vi "p2.vi"() -> ()   [LabVIEW 2021, in "d9.lvlib"]
uses:
  d9.lvlib
  939e70a1-15eb-480c-88e0-20e72bed207b.vi
  AOC/AOC.lvlib
panel:
  in  "Defer Panel Updates":bool=TRUE
  in  "Move Delay":u32
  out "Moves Remaining":i32
  out "Rope":cluster{"x":i64, "y":i64}[](graph)
  in  "Example":string="R 5\nU 8\nL 8\nD 3\nR 17\nD 10\nL 25\nU 20"
  in  "Example":bool=TRUE
  out "Answer":i32=36
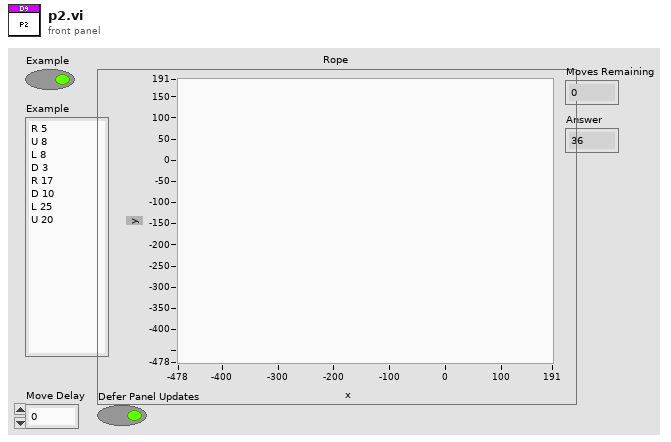
[diagram p1: front panel]
diagram:
  w3 = -10.0 ("X Scale.Range:Minimum")
  w4 = 10.0 ("X Scale.Range:Maximum")
  w8 = 10 ("dimension size")
  n1 = control-ref of="Rope"() -> (w6:refnum<vi>)
  n2 = property on="Property Node" class="XYGraph (strict)"(reference=w6, "XScale.Maximum"=w4, "YScale.Maximum"=w4, "XScale.Minimum"=w3, "YScale.Minimum"=w3) -> (reference out=w5:refnum<vi>)  [unwired: 1 in, 1 out]
  n3 = call "Get Input.vi"() -> ()  [unwired: 11 in, 1 out]
  n4 = Select(t="Example", s="Example", f="R 1\nU 2\nR 1\nL 2\nD 2\nU 1\nR 2\nU 1\nL 2\nU 1\nD 2\nR 1\nD 1\nL 1\nU 2\nD 2\nL 2\nD 1\nU 2\nD 2\nL 1\nU 1\nL 2\nD 2\nU 2\nL 1\nU 2\nL 1\nR 2\nU 1\nL 1\nR 2\nD 1\nU 2\nR 1\nU 1\nR 2\nU 1\nR 2\nU 1\nD 1\nU 1\nD 1\nL 2\nD 2\nR 1\nU 1\nR 1\nU 1\nL 1\nU 1\nD 2\nR 2\nD 2\nL 2\nU 2\nR 1\nD 1\nU 1\nD 2\nR 1\nD 2\nL 2\nR 2\nL 1\nU 1\nL 2\nD 2\nL 2\nD 1\nR 1\nL 2\nD 2\nR 1\nL 1\nR 1\nD 1\nR 1\nD 2\nL 2\nU 1\nD 2\nR 2\nD 1\nU 1\nL 1\nD 1\nU 2\nR 1\nU 1\nL 2\nU 1\nL 1\nU 2\nL 2\nD 2\nU 1\nL 1\nU 2\nD 2\nL 2\nD 2\nR 2\nU 2\nL 2\nD 1\nU 1\nR 2\nD 2\nL 2\nR 2\nD 2\nL 1\nD 1\nU 2\nR 2\nD 3\nR 1\nU 3\nL 3\nD 2\nR 1\nD 1\nL 2\nD 1\nR 2\nU 3\nL 2\nU 2\nR 3\nU 3\nL 1\nD 3\nR 3\nU 2\nR 3\nU 3\nL 1\nD 3\nR 3\nL 2\nR 2\nL 3\nD 3\nR 2\nD 2\nR 2\nD 1\nR 1\nL 1\nD 2\nR 1\nD 2\nU 1\nR 2\nL 2\nR 2\nU 2\nR 2\nD 1\nU 1\nD 1\nL 3\nU 3\nD 3\nL 1\nU 2\nR 2\nU 2\nR 1\nU 1\nL 2\nU 2\nR 3\nU 1\nD 3\nR 3\nU 2\nR 1\nU 1\nD 3\nL 2\nU 3\nL 1\nR 2\nD 3\nR 2\nU 1\nR 2\nD 1\nU 3\nL 2\nD 1\nR 1\nL 3\nR 3\nD 2\nR 1\nU 2\nR 3\nD 2\nU 2\nL 2\nU 1\nR 2\nU 2\nL 2\nD 3\nL 2\nD 1\nL 1\nU 2\nL 1\nD 2\nR 1\nD 2\nR 1\nL 2\nU 1\nL 1\nU 1\nD 2\nR 4\nD 4\nL 2\nR 4\nD 1\nL 2\nD 2\nL 4\nU 4\nD 4\nL 3\nR 3\nD 1\nL 1\nD 1\nU 4\nR 4\nU 4\nD 2\nR 1\nU 3\nR 2\nU 3\nR 4\nD 3\nU 3\nL 4\nD 1\nR 2\nU 3\nD 4\nU 3\nR 2\nL 1\nD 2\nU 2\nR 3\nU 2\nR 2\nD 2\nL 2\nU 4\nR 1\nL 3\nR 1\nL 1\nD 3\nR 4\nD 2\nR 4\nU 3\nL 1\nD 1\nR 4\nU 3\nD 1\nL 3\nR 1\nL 3\nD 2\nL 2\nR 3\nL 4\nD 4\nU 1\nL 1\nR 1\nD 3\nL 2\nR 1\nD 3\nR 2\nD 4\nU 4\nR 3\nU 1\nD 3\nL 3\nD 3\nU 1\nD 2\nU 4\nR 4\nU 2\nD 1\nR 1\nD 4\nL 2\nR 3\nU 4\nL 1\nD 1\nU 4\nL 3\nD 4\nU 2\nR 4\nU 2\nR 4\nU 2\nL 1\nR 1\nL 3\nD 4\nL 2\nR 2\nL 3\nU 3\nR 4\nL 2\nR 1\nD 5\nU 1\nR 1\nU 2\nR 1\nU 4\nL 3\nU 4\nR 2\nD 3\nL 4\nR 3\nL 2\nU 2\nR 1\nL 3\nD 5\nR 3\nL 2\nU 5\nR 2\nU 5\nL 5\nU 4\nR 4\nD 2\nR 4\nD 3\nR 2\nD 3\nU 2\nL 3\nD 3\nL 1\nU 4\nD 3\nL 1\nD 1\nR 2\nL 4\nR 3\nU 1\nR 3\nL 2\nR 3\nD 4\nR 2\nU 3\nL 4\nR 5\nL 1\nU 1\nD 5\nU 2\nR 5\nL 4\nD 3\nL 1\nD 3\nU 1\nR 2\nD 1\nL 5\nD 2\nR 4\nL 1\nD 2\nR 4\nL 3\nR 3\nL 3\nR 4\nL 3\nU 3\nD 4\nU 2\nR 1\nD 1\nU 1\nR 5\nD 5\nL 5\nR 3\nU 2\nD 4\nL 5\nD 1\nL 4\nR 4\nU 2\nL 2\nR 2\nU 3\nL 1\nU 3\nL 1\nD 4\nU 5\nD 5\nR 4\nL 4\nR 5\nD 4\nU 5\nL 4\nU 1\nD 4\nR 5\nD 2\nU 4\nR 2\nU 3\nD 2\nU 6\nD 4\nR 1\nD 4\nR 3\nL 1\nR 5\nU 6\nD 5\nL 4\nR 3\nL 4\nR 5\nD 1\nR 3\nD 2\nL 6\nU 5\nR 6\nL 2\nD 6\nU 1\nL 3\nD 4\nR 6\nD 3\nL 3\nR 5\nU 6\nD 5\nU 1\nR 4\nL 4\nU 4\nR 5\nD 1\nL 4\nU 6\nL 2\nR 3\nL 2\nR 3\nL 3\nR 4\nU 3\nD 1\nR 6\nD 5\nL 2\nR 4\nU 4\nD 2\nL 1\nR 2\nD 3\nL 4\nD 4\nR 4\nD 6\nR 1\nL 2\nR 5\nD 3\nU 5\nR 4\nL 6\nD 6\nU 4\nR 4\nL 4\nU 4\nR 5\nD 1\nU 1\nR 4\nL 2\nU 6\nD 3\nL 3\nU 6\nD 1\nU 4\nD 6\nR 6\nU 1\nR 2\nU 5\nD 4\nL 2\nU 5\nD 1\nL 5\nU 1\nR 3\nD 2\nR 1\nL 3\nD 1\nR 1\nL 2\nR 6\nD 6\nR 4\nU 4\nL 5\nR 6\nL 5\nR 4\nD 3\nL 2\nR 4\nL 2\nU 6\nD 5\nR 1\nL 3\nR 1\nU 2\nR 6\nL 2\nD 7\nL 2\nD 4\nR 2\nU 6\nD 4\nR 5\nU 6\nR 3\nL 3\nU 2\nR 3\nU 1\nR 7\nU 2\nR 2\nD 7\nR 1\nU 5\nD 1\nL 5\nU 5\nR 2\nD 5\nR 4\nU 5\nL 3\nD 4\nL 6\nR 7\nL 2\nD 3\nL 2\nD 6\nU 6\nL 1\nD 7\nU 6\nL 7\nR 5\nL 1\nU 7\nR 1\nL 4\nR 4\nL 5\nU 7\nD 4\nR 7\nL 5\nU 7\nL 6\nU 3\nD 5\nR 5\nU 7\nR 5\nL 3\nU 6\nR 2\nU 3\nR 3\nU 6\nL 5\nD 6\nL 4\nD 5\nR 1\nL 3\nU 6\nR 6\nU 6\nL 1\nD 2\nL 5\nD 1\nL 6\nU 5\nD 5\nR 5\nD 6\nL 4\nU 5\nR 2\nU 4\nD 7\nL 1\nU 1\nD 1\nL 1\nD 4\nU 1\nL 6\nU 1\nR 5\nD 1\nU 1\nR 1\nU 5\nR 4\nU 5\nL 2\nU 6\nL 7\nR 2\nU 4\nR 5\nL 1\nR 8\nL 2\nD 7\nR 7\nD 2\nL 2\nR 2\nD 2\nU 7\nD 7\nR 4\nU 1\nR 2\nL 6\nU 1\nL 3\nU 2\nD 7\nR 6\nL 5\nD 1\nL 3\nU 6\nD 2\nU 2\nR 4\nD 1\nL 7\nU 3\nD 8\nU 4\nD 8\nL 8\nU 6\nL 3\nU 4\nR 4\nU 8\nD 1\nR 7\nU 5\nL 8\nU 4\nL 4\nD 7\nU 8\nL 2\nD 8\nL 1\nR 1\nL 1\nR 8\nL 8\nR 5\nL 1\nR 4\nD 3\nR 2\nU 8\nL 6\nR 4\nL 3\nR 8\nL 4\nD 5\nR 3\nU 2\nD 8\nU 4\nR 6\nD 4\nR 3\nL 7\nD 8\nL 2\nU 6\nD 7\nR 3\nL 5\nR 4\nD 3\nL 4\nR 8\nL 7\nD 8\nR 3\nU 3\nL 3\nR 6\nL 1\nU 3\nL 1\nU 4\nR 8\nL 8\nR 2\nD 3\nL 2\nR 1\nD 2\nR 6\nU 3\nD 1\nU 3\nR 1\nU 2\nR 2\nL 2\nD 6\nU 7\nL 8\nD 6\nU 2\nR 3\nL 6\nU 9\nD 6\nU 1\nD 3\nU 4\nR 3\nL 9\nD 6\nU 9\nD 1\nL 5\nU 5\nD 6\nU 4\nL 8\nU 8\nD 3\nL 3\nU 9\nR 5\nL 7\nD 1\nR 9\nU 8\nD 1\nR 1\nU 9\nD 4\nR 6\nU 8\nR 6\nU 3\nD 2\nU 8\nL 8\nU 9\nD 4\nL 3\nU 4\nD 3\nL 9\nR 7\nL 9\nR 3\nL 5\nD 7\nL 8\nU 9\nL 7\nD 1\nL 6\nU 7\nL 6\nD 8\nU 9\nL 7\nR 7\nD 1\nR 6\nD 4\nU 7\nR 7\nL 8\nD 4\nR 1\nL 7\nD 2\nU 3\nD 1\nR 7\nD 7\nR 7\nL 6\nD 9\nU 7\nD 5\nR 7\nL 1\nR 9\nU 1\nL 2\nU 5\nR 4\nD 7\nR 2\nD 5\nU 4\nD 3\nR 9\nU 2\nD 9\nU 1\nR 9\nU 9\nD 1\nL 7\nU 6\nD 6\nU 9\nL 5\nU 2\nD 6\nL 4\nD 3\nU 1\nR 2\nL 1\nR 1\nD 1\nR 1\nU 1\nR 4\nL 7\nR 2\nD 1\nU 3\nD 3\nR 10\nL 7\nR 7\nD 2\nL 6\nR 9\nU 9\nD 8\nU 9\nR 2\nU 6\nD 9\nU 1\nL 2\nR 10\nL 9\nR 10\nL 6\nR 4\nD 4\nR 4\nU 4\nD 4\nL 5\nR 8\nD 4\nL 7\nD 6\nL 8\nR 9\nL 8\nD 7\nR 2\nU 2\nD 5\nL 4\nR 8\nD 7\nR 6\nD 7\nL 5\nU 7\nR 1\nD 7\nR 9\nD 5\nU 3\nL 8\nD 7\nU 4\nD 4\nR 10\nU 7\nD 4\nU 2\nR 7\nL 4\nU 2\nD 9\nL 5\nR 2\nU 10\nL 9\nR 10\nL 1\nD 5\nR 10\nL 5\nR 5\nD 5\nR 10\nL 4\nU 9\nD 7\nR 10\nL 6\nU 3\nD 5\nU 6\nL 6\nU 10\nL 1\nU 10\nD 4\nL 7\nU 2\nL 10\nR 4\nL 7\nR 4\nD 10\nL 4\nU 10\nL 10\nD 9\nU 4\nR 8\nU 8\nR 5\nU 3\nD 10\nR 7\nL 10\nR 9\nL 1\nD 6\nL 11\nD 11\nR 3\nL 8\nU 6\nR 9\nD 5\nR 9\nD 4\nU 7\nD 4\nR 4\nU 10\nD 4\nR 2\nL 3\nU 5\nD 11\nR 8\nL 8\nU 7\nR 3\nD 8\nU 5\nR 10\nD 5\nR 2\nU 11\nD 10\nR 1\nU 9\nL 10\nR 2\nD 11\nR 6\nL 3\nR 10\nU 2\nD 6\nL 10\nU 5\nL 6\nU 1\nR 10\nU 8\nR 8\nD 4\nU 8\nL 11\nR 7\nL 2\nD 2\nR 5\nU 10\nL 3\nR 6\nL 8\nR 8\nU 8\nD 3\nL 7\nR 5\nL 6\nD 11\nL 6\nD 7\nU 6\nD 3\nU 9\nL 7\nR 8\nL 3\nR 10\nD 11\nL 11\nR 4\nD 6\nL 7\nD 9\nR 10\nU 11\nL 9\nD 8\nL 2\nU 1\nD 7\nU 10\nD 11\nR 5\nD 11\nL 6\nD 5\nR 6\nD 5\nR 11\nU 3\nD 6\nR 5\nU 7\nD 2\nR 6\nU 5\nD 9\nU 3\nR 7\nD 10\nU 5\nD 4\nR 6\nU 11\nL 10\nU 5\nL 6\nR 5\nU 7\nL 7\nR 5\nD 9\nU 11\nL 7\nU 8\nL 7\nU 3\nL 8\nR 10\nU 11\nR 8\nL 12\nU 8\nD 2\nL 2\nD 2\nU 10\nR 11\nU 2\nR 6\nU 3\nD 9\nU 5\nD 12\nL 11\nD 8\nU 12\nR 4\nU 1\nL 2\nR 10\nD 6\nL 10\nU 2\nR 4\nL 4\nD 8\nU 9\nL 4\nD 10\nU 5\nR 10\nL 2\nD 2\nU 2\nR 7\nD 8\nR 1\nU 11\nD 1\nL 7\nR 12\nD 12\nR 3\nL 11\nR 10\nU 11\nR 5\nD 6\nR 11\nD 2\nL 3\nD 12\nL 9\nR 6\nU 1\nD 2\nR 6\nD 5\nU 7\nR 2\nD 5\nU 3\nD 12\nR 12\nL 9\nR 9\nD 12\nR 8\nD 11\nL 7\nU 4\nD 11\nR 1\nU 9\nL 1\nD 2\nR 3\nU 1\nD 1\nR 2\nD 11\nU 12\nR 7\nD 1\nU 13\nL 5\nD 13\nL 10\nD 12\nL 7\nD 9\nL 7\nU 6\nL 1\nR 1\nL 10\nR 7\nL 6\nU 7\nR 10\nU 7\nR 11\nU 12\nL 2\nD 11\nL 5\nU 2\nD 8\nL 10\nD 13\nU 10\nL 9\nU 5\nD 11\nR 6\nL 9\nR 2\nL 6\nU 4\nR 7\nD 11\nL 3\nU 6\nD 13\nU 2\nR 13\nU 11\nL 12\nD 13\nL 1\nR 9\nD 10\nU 6\nL 13\nU 2\nL 12\nD 7\nR 1\nL 6\nD 1\nU 10\nD 5\nL 2\nU 12\nR 1\nU 9\nD 4\nU 10\nL 1\nR 1\nU 8\nR 2\nD 1\nL 6\nU 11\nD 2\nU 7\nD 11\nU 9\nD 6\nU 5\nD 13\nR 2\nU 8\nL 4\nU 4\nR 2\nU 1\nD 3\nL 1\nD 13\nR 9\nL 4\nD 5\nL 7\nU 2\nD 10\nL 6\nU 11\nD 1\nU 5\nR 4\nD 9\nR 12\nD 2\nU 9\nL 10\nU 6\nD 2\nL 8\nU 4\nL 4\nD 12\nU 3\nL 14\nD 12\nR 12\nL 7\nU 5\nL 2\nD 4\nL 13\nD 10\nL 8\nD 12\nR 13\nU 8\nD 14\nU 4\nR 11\nL 4\nR 13\nL 2\nU 1\nD 10\nL 12\nD 13\nL 4\nD 11\nR 14\nU 8\nL 11\nD 2\nU 8\nL 8\nD 3\nL 14\nU 7\nL 2\nR 2\nD 6\nU 1\nL 12\nR 12\nU 4\nL 1\nU 13\nR 12\nD 8\nU 10\nR 2\nL 7\nR 4\nD 4\nL 14\nU 2\nD 2\nU 11\nL 7\nR 12\nU 9\nL 11\nR 6\nD 6\nR 8\nL 1\nD 9\nL 7\nD 10\nR 6\nD 6\nL 5\nD 14\nL 12\nU 12\nR 4\nD 14\nL 10\nD 11\nL 3\nD 3\nU 9\nL 6\nD 10\nU 1\nL 10\nD 9\nR 8\nL 3\nU 7\nR 4\nU 9\nL 5\nR 7\nD 7\nL 5\nU 4\nR 4\nL 7\nR 8\nL 2\nR 5\nL 10\nR 2\nL 12\nD 12\nL 6\nR 4\nL 11\nD 13\nL 13\nR 10\nD 12\nU 5\nR 11\nL 15\nR 6\nU 9\nD 5\nU 6\nL 1\nD 1\nR 7\nD 5\nR 15\nU 11\nR 5\nD 15\nR 13\nU 8\nR 11\nU 7\nD 4\nL 6\nD 11\nU 1\nL 2\nR 11\nL 12\nD 5\nR 3\nL 14\nR 15\nL 14\nU 13\nD 9\nL 3\nD 4\nU 9\nL 3\nR 14\nU 3\nR 15\nL 14\nR 4\nU 15\nL 1\nD 11\nL 13\nD 14\nL 1\nD 1\nU 13\nD 7\nU 13\nD 15\nU 15\nL 6\nD 7\nR 15\nL 10\nU 6\nR 7\nL 13\nU 3\nD 9\nL 3\nD 10\nR 14\nD 15\nL 6\nD 4\nU 11\nL 11\nD 6\nU 8\nD 15\nR 5\nL 9\nD 15\nU 15\nR 9\nD 11\nU 7\nL 9\nU 8\nD 2\nL 4\nD 11\nU 12\nR 11\nU 5\nL 12\nU 5\nR 14\nL 10\nR 6\nD 3\nL 13\nU 6\nR 10\nD 10\nU 9\nD 3\nR 7\nL 13\nR 15\nU 6\nL 13\nU 11\nD 9\nL 7\nR 8\nU 6\nR 12\nU 2\nL 8\nU 10\nD 11\nU 14\nR 3\nL 15\nU 9\nL 2\nU 2\nD 11\nL 11\nR 3\nD 14\nU 3\nL 1\nU 2\nD 12\nL 5\nR 5\nD 10\nL 16\nR 4\nU 3\nL 6\nR 9\nL 7\nR 2\nU 15\nR 6\nL 12\nD 16\nL 16\nD 15\nU 12\nL 6\nD 9\nU 8\nL 10\nD 11\nU 4\nD 12\nU 7\nD 14\nU 1\nD 10\nR 10\nD 14\nL 5\nD 6\nR 8\nL 16\nU 7\nL 12\nR 13\nL 11\nD 12\nR 5\nD 11\nL 5\nR 4\nD 15\nL 13\nD 10\nR 2\nL 16\nD 14\nR 15\nD 11\nU 2\nD 12\nL 11\nD 1\nR 5\nD 6\nU 13\nL 10\nR 1\nU 10\nD 12\nL 10\nD 10\nR 11\nL 10\nD 11\nL 3\nR 11\nD 12\nL 6\nU 2\nL 10\nD 9\nL 11\nU 12\nD 14\nL 6\nU 16\nD 2\nL 2\nD 14\nU 7\nR 12\nD 14\nL 4\nU 3\nR 16\nD 2\nL 5\nR 10\nL 1\nR 11\nL 14\nD 3\nL 17\nD 4\nU 1\nR 8\nD 8\nL 5\nU 1\nL 13\nD 15\nU 17\nL 1\nD 14\nU 4\nR 1\nU 2\nD 14\nR 10\nU 14\nD 17\nR 10\nU 13\nD 12\nU 8\nL 11\nU 17\nR 12\nU 6\nD 8\nR 10\nU 16\nD 4\nR 3\nD 3\nU 4\nL 3\nU 5\nR 16\nL 5\nR 16\nD 17\nR 12\nL 11\nR 13\nU 12\nL 8\nR 5\nD 6\nU 16\nL 16\nD 2\nL 11\nD 1\nR 1\nD 14\nR 15\nL 6\nU 14\nR 12\nD 11\nL 9\nU 6\nL 11\nD 15\nU 17\nL 1\nU 3\nL 6\nU 5\nR 16\nL 14\nR 9\nL 12\nD 14\nU 13\nL 3\nU 13\nD 7\nR 2\nU 7\nD 5\nL 17\nD 6\nL 16\nR 5\nD 4\nR 3\nU 11\nD 3\nU 9\nD 10\nU 2\nL 6\nD 6\nR 15\nD 17\nR 1\nL 15\nD 2\nU 5\nR 2\nD 6\nL 8\nR 5\nL 2\nD 17\nU 9\nD 9\nL 7\nR 12\nL 12\nR 18\nL 10\nR 9\nD 6\nR 9\nU 15\nL 17\nD 18\nR 1\nL 15\nD 4\nR 6\nU 3\nR 6\nU 3\nD 1\nU 9\nD 8\nR 3\nD 6\nU 3\nR 8\nL 8\nR 10\nU 7\nD 16\nU 17\nR 11\nU 8\nD 1\nU 8\nL 4\nR 12\nD 10\nU 7\nD 18\nU 7\nD 12\nL 18\nU 9\nR 2\nU 5\nD 14\nR 13\nD 15\nU 17\nD 16\nL 4\nD 10\nL 2\nU 7\nL 7\nD 13\nR 13\nU 12\nR 16\nU 17\nR 3\nU 12\nR 6\nD 12\nU 11\nL 6\nU 15\nL 12\nR 1\nD 6\nL 16\nR 1\nD 7\nR 17\nL 15\nD 15\nU 9\nR 18\nD 13\nR 14\nD 1\nR 1\nD 16\nL 18\nR 1\nU 14\nL 8\nD 14\nR 15\nD 2\nU 10\nD 17\nU 3\nD 9\nR 7\nD 17\nU 3\nD 15\nL 17\nD 17\nR 1\nD 10\nL 9\nD 14\nR 5\nU 14\nR 14\nD 12\nR 18\nU 4\nD 2\nU 17\nD 12\nL 4\nU 9\nL 9\nU 17\nR 4\nU 17\nR 8\nD 10\nR 3\nD 9\nU 17\nL 5\nR 16\nU 9\nL 5\nD 15\nU 2\nD 7\nL 15\nU 1\nL 16\nR 8\nL 13\nR 3\nD 8\nR 1\nD 8\nL 10\nU 16\nR 16\nL 2\nU 3\nD 9\nU 12\nD 1\nL 10\nD 15\nU 7\nR 3\nD 15\nU 4\nL 6\nR 14\nU 13\nR 16\nU 2\nR 9\nU 15\nD 8\nL 8\nR 17\nD 3\nL 17\nD 13\nU 8\nD 11\nR 13\nL 3\nD 2\nU 14\nR 1\nU 10\nR 11\nD 16\nL 10\nR 17\nU 7\nL 13\nR 3\nL 18\nR 5\nU 7\nL 12\nD 4\nU 5\nL 17\nR 18\nL 4\nR 19\nL 12\nU 17\nR 2\nL 11\nR 9\nD 16\nR 19\nL 18\nU 11\nD 4\nR 13\nL 18\nU 13\nR 19\nD 3\nR 10\nL 3\nR 5\nD 2\nR 2\nL 18\nD 15\nR 19\nL 5\nD 4\nU 5\nR 12\nD 15\nL 13\nR 16\nU 16\nL 6\nU 12\nL 8") -> (s? t:f=w20:string)
  n5 = property class="VI"() -> ("Panel"=w2:refnum<vi>)  [unwired: 2 in, 2 out]
  n6 = call <vilib>:"Delimited String to 1D String Array.vi"("delimiter"="\n", "delimited string"=w20) -> ("string array"=w10:string[])  [unwired: 9 in]
  n7 = Initialize Array(cluster{"x":i64, "y":i64} {"x"=0, "y"=0} ("Knot"), w8) -> (w11:cluster{"x":i64, "y":i64}[])
  n8 = Decrement(x=w8) -> (x-1=w7:i32)
  n9 = for {
    N -> [w30]
    tunnel: w10 -> [w42] mode=indexing
    shift-right: [w33] -> _
    shift-left: w11 -> [w38]
    tunnel: [w37] -> w16 mode=concatenating
    tunnel: w7 -> [w34]
    tunnel: w5 -> [w32]
    tunnel: w2 -> [w27]
    i -> [w31]
    n10 = call <vilib>:"Space Constant.vi"() -> ("String"=w41:string)
    n11 = property class="Pnl"(reference=w27, "Defer Panel Updates"="Defer Panel Updates") -> (reference out=w26:refnum<vi>, error out=w24:errorcluster)  [unwired: 1 in]
    n12 = Increment(x=w31) -> (x+1=w29:i32)
    n13 = call <vilib>:"Delimited String to 1D String Array.vi"("delimiter"=w41, "delimited string"=w42) -> ("string array"=w40:string[])  [unwired: 9 in]
    n14 = Subtract(x=w30, y=w29) -> (x-y=→"Moves Remaining":i32)
    n15 = Index Array(array=w40) -> (element #1=w39:string, element #2=w36:string)  [unwired: 2 in]
    n16 = Decimal String To Number(string=w36) -> (number=w35:i32)  [unwired: 2 in, 1 out]
    n17 = for {
      N: w35 -> [_]
      tunnel: w39 -> [w51]
      tunnel: [w50] -> w37 mode=indexing
      shift-right: [w44] -> w33
      shift-left: w38 -> [w52]
      tunnel: w34 -> [w43]
      tunnel: w32 -> [w49]
      tunnel: "Move Delay" -> [w47]
      tunnel: w24 -> [w46]
      tunnel: [w46] -> w23
      n18 = call "Move Head.vi"("Move Delay"=w47, "XYGraph in"=w49, "Direction"=w51, "Rope in"=w52) -> ("Rope out"=w53:cluster{"x":i64, "y":i64}[], "XY Graph out"=w48:refnum<vi>)  [unwired: 6 in]
      n19 = call "Move Tail.vi"("Move Delay"=w47, "XYGraph in"=w48, "Rope in"=w53) -> ("Rope out"=w45:cluster{"x":i64, "y":i64}[])  [unwired: 7 in, 1 out]
      n20 = in-place {
        in-place-border: [w54] -> w50
        n21 = in-place-array #1(w45, w43) -> (w54:cluster{"x":i64, "y":i64})
        n22 = in-place-array #1(w54) -> (w44:cluster{"x":i64, "y":i64}[])  [unwired: 1 out]
      }
    }
    n23 = property class="Pnl"(reference=w26, error in=w23, "Defer Panel Updates"=FALSE) -> ()  [unwired: 2 out]
  }
  n24 = Build Array (concatenate)(w16, cluster{"x":i64, "y":i64} {"x"=0, "y"=0} ("element")) -> (w14:cluster{"x":i64, "y":i64}[])
  n25 = call "Remove Duplicates From 1D Array.vim"("array"=w14) -> ("array with duplicates removed"=w13:cluster{"x":i64, "y":i64}[])  [unwired: 10 in]
  n26 = Array Size(array=w13) -> (size(s)=→"Answer":i32)
